vi "Get Target.vi"(7 "index":i32, 8 "error in":errorcluster, 11 "Builder in":refnum<class "Builder.lvclass">) -> (0 "error out":errorcluster, 1 "Build Object type":T1, 2 "element":refnum<vi>, 3 "Builder out":refnum<class "Builder.lvclass">)   [LabVIEW 2021, in "App-Builder Library.lvlib" / "Builder.lvclass"]
uses:
  Builder.lvclass
  Build object type.ctl
  Builder.lvclass/Builder.ctl
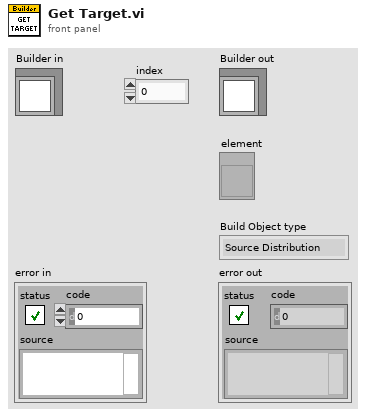
[diagram p1: front panel]
types:
  T1 = typedef "App-Builder Library.lvlib/Builder.lvclass/Build object type.ctl" = enum16{"Source Distribution", "Deployable Source Distribution", "DLL", "EXE", "Packed Library", "Deployable Packed", "RT EXE", ".NET Interop Assembly"}
  T2 = typedef "App-Builder Library.lvlib/Builder.lvclass/Build specification.ctl" = cluster{"target name":string, "Build specification":string, "Project Path":path, "Build Object type":T1}
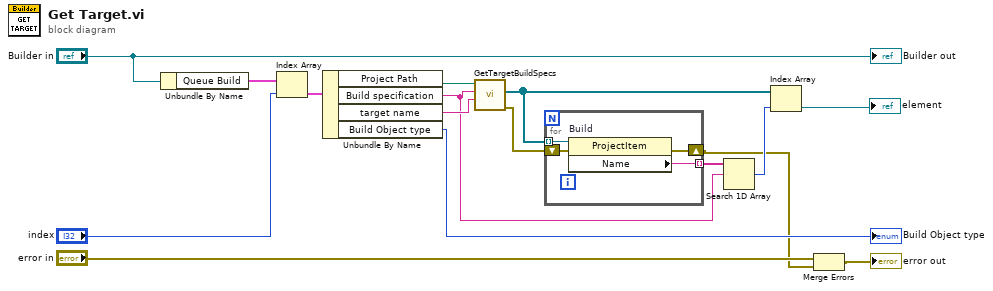
[diagram p0: block diagram]
diagram:
  n1 = Unbundle By Name("Builder in") -> ("Queue Build"=w10:T2[])
  n2 = Index Array(array=w10, index="index") -> (element=w11:T2)
  n3 = Unbundle By Name(w11) -> ("Project Path"=w12:path, "Build specification"=w5:string, "target name"=w8:string, "Build Object type"=→"Build Object type":T1)
  n4 = call <vilib>:"GetTargetBuildSpecs.vi"("Name of target (My Computer)"=w8, "Name of build specification (if empty: get all)"=w5, "Path to project"=w12) -> ("error out"=w6:errorcluster, "buildspec refs"=w4:refnum<vi>[])  [unwired: 6 in, 1 out]
  n5 = for {
    tunnel: w4 -> [w20] mode=indexing
    tunnel: [w19] -> w7 mode=indexing
    shift-right: [w17] -> w2
    shift-left: w6 -> [w18]
    n6 = property on="Build" class="ProjectItem"(reference=w20, error in=w18) -> (error out=w17:errorcluster, "Name"=w19:string)  [unwired: 1 out]
  }
  n7 = Search 1D Array(1D array=w7, element=w5) -> (index of element=w3:i32)  [unwired: 1 in]
  n8 = Index Array(array=w4, index=w3) -> (element=→"element":refnum<vi>)
  n9 = Merge Errors("error in", w2) -> (→"error out":errorcluster)
  "Builder out" <- "Builder in"
